vi "Login.vi"(4 "Source (\"\")":string, 6 "User ID (\"\")":string, 7 "Function Name (0 : Setting)":i32(ring) items=["Setting", "Monitor"], 8 "error in (no error)":errorcluster, 9 "Password (\"\")":string, 10 "User Name (\"admin\")":string="admin", 11 "VISA resource name":refnum<visa-resource-name>) -> (0 "error out":errorcluster, 3 "VISA resource name out":refnum<visa-resource-name>)   [LabVIEW 2011, in "Yokogawa DX Series.lvlib"]
doc: "This VI logs in the instrument.\nSpecified user name provides access authority as follows,\n\nAdministrator:\n An administrator has the whole authority.\n\nUser:\n A user has limited authority to use. \n The user can read settings but cannot change settings. \n The user can output the measurement data."
uses:
  <instrlib>/Yokogawa DX Series/Yokogawa DX Series.lvlib
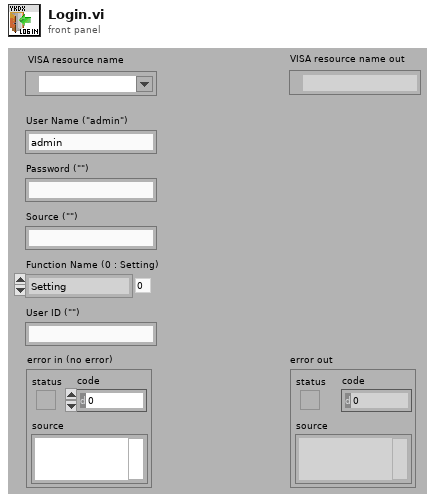
[diagram p1: front panel]
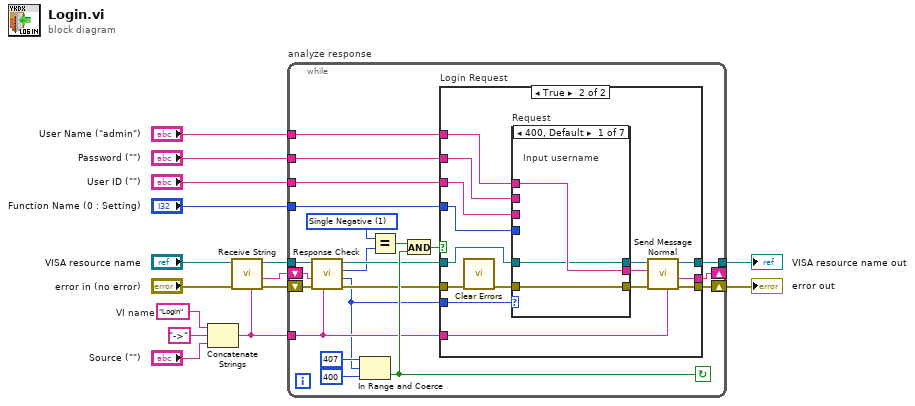
[diagram p0: block diagram]
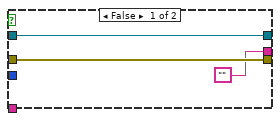
[diagram p2: hidden frame]
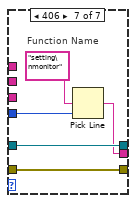
[diagram p8: hidden frame]
diagram:
  w15 = "Login"  # VI name
  n1 = Concatenate Strings(w15, "->", "Source (\"\")") -> (w8:string)
  n2 = call <instrlib>:"Receive String.vi"("Source (\"\")"=w8, "error in (no error)"="error in (no error)", "VISA resource name"="VISA resource name") -> ("error out"=w7:errorcluster, "Read Buffer"=w6:string, "VISA resource name out"=w5:refnum<visa-resource-name>)  [unwired: 1 in, 5 out]
  n3 = while "analyze response" {
    shift-left: w7 -> [w26]
    shift-right: [w34] -> w11
    tunnel: w8 -> [w25]
    shift-left: w6 -> [w27]
    shift-right: [w32] -> _
    tunnel: "Password (\"\")" -> [w19]
    tunnel: "User Name (\"admin\")" -> [w20]
    tunnel: "User ID (\"\")" -> [w18]
    tunnel: "Function Name (0 : Setting)" -> [w17]
    tunnel: w5 -> [w28]
    tunnel: [w33] -> w12
    stop <- w29 continue-if-true
    w16 = 1 items=["Affirmative", "Single Negative", "Multiple Negative", "ASCII", "Binary", "End"] ("Response Type")
    n4 = call <instrlib>:"Response Check.vi"("Source (\"\")"=w25, "error in (no error)"=w26, "Message In (\"\")"=w27, "VISA resource name"=w28) -> ("error out"=w24:errorcluster, "Internal Error Number"=w21:i32, "Response Type"=w22:i32, "VISA resource name out"=w23:refnum<visa-resource-name>)  [unwired: 4 out]
    n5 = In Range and Coerce(upper limit=407, x=w21, lower limit=400) -> (In Range?=w29:bool)  [unwired: 1 out]
    n6 = Equal?(x=w16, y=w22) -> (x = y?=w36:bool)
    n7 = And(x=w36, y=w29) -> (x .and. y?=w35:bool)
    n8 = case "Login Request" shown="True" w35 {
      tunnel: w19 -> [_ w54]
      tunnel: w20 -> [_ w53]
      tunnel: w25 -> [_ w42]
      tunnel: w23 -> [w39 w50]
      tunnel: w24 -> [w38 w52]
      tunnel: [w38 w47] -> w34
      tunnel: [w39 w48] -> w33
      tunnel: w21 -> [_ w49]
      tunnel: ["" w46] -> w32
      tunnel: w18 -> [_ w41]
      tunnel: w17 -> [_ w40]
      frame False {
      }
      frame True {
        n9 = call <vilib>:"Clear Errors.vi"("error in (no error)"=w52) -> ("error out"=w51:errorcluster)  [unwired: 6 out]
        n10 = case "Request" shown="400, Default" w49 {
          tunnel: w53 -> [w56 _ w62 w65 w68 _ _]
          tunnel: w54 -> [_ w59 _ _ _ _ _]
          tunnel: w51 -> [w57 w60 w63 w66 w69 w72 w77]
          tunnel: [w57 w60 w63 w66 w69 w72 w77] -> w43
          tunnel: [w56 w59 w62 w65 w68 w70 w74] -> w45
          tunnel: w50 -> [w55 w58 w61 w64 w67 w71 w76]
          tunnel: [w55 w58 w61 w64 w67 w71 w76] -> w44
          tunnel: w41 -> [_ _ _ _ _ w70 _]
          tunnel: w40 -> [_ _ _ _ _ _ w75]
          frame 400, Default {
            # "Input username"
          }
          frame 401 {
            # "Input password"
          }
          frame 402 {
            # "admin or user"
          }
          frame 403 {
            # "try again"
          }
          frame 404 {
            # "try again"
          }
          frame 405 {
            # "user ID"
          }
          frame 406 {
            # "Function Name"
            n11 = Pick Line(multi-line string="setting\nmonitor", line index=w75) -> (output string=w74:string)  [unwired: 1 out]
          }
        }
        n12 = call <instrlib>:"Send Message Normal.vi"("Source (\"\")"=w42, "error in (no error)"=w43, "Send Message (\"\")"=w45, "VISA resource name"=w44) -> ("error out"=w47:errorcluster, "Read Buffer"=w46:string, "VISA resource name out"=w48:refnum<visa-resource-name>)  [unwired: 1 in, 4 out]
      }
    }
  }
  "error out" <- w11
  "VISA resource name out" <- w12
